vi "RTK-Make Child.vi"(1 "error in (no error)":errorcluster, 2 "Window Number":i32, 3 "Name of Parent Panel":string) -> (0 "error out":errorcluster)   [LabVIEW 2021]
doc: "Developer: Wayne Lootsma\nDate: 01/08/2003\nDescription:\nVi from NIs website for making an IMAQ window a child window, works only on Windows systems. Here is the original text:\nIMAQ MakeChild will allow you to embed your IMAQ Vision display into any vi's Front Panel.\n\nIt is okay to use IMAQ WindMove, IMAQ WindSize, IMAQ WindSetup, etc to define properties of the child window before calling this function. Doing so will allow you to customize the look and feel of your user interface.\n\nParent Panel Name is the name of the vi into which the IMAQ Vision window is to be embedded. This vi must be loaded into memory. \n\nWindow Number is the IMAQ Vision window number of the window which is to be made a child. This number is specified in IMAQ Create. \n\n\nDialog Panel: False\nGUI Panel: False\n\nDLL Description:\nInterface with a window for an IMAQ window.\n\nParty's Responsible: Microsoft Corp.\nDLL Filename: User32.dll\nDLL Location: C:\\Windows\\System\nProduct Name, Compiler and Version Number: Microsoft Visual C++, C Compiler V 2.0\nOperating System: Windows NT, 2000.\nLast Date Modified: 03/26/2003"
uses:
  User32.dll
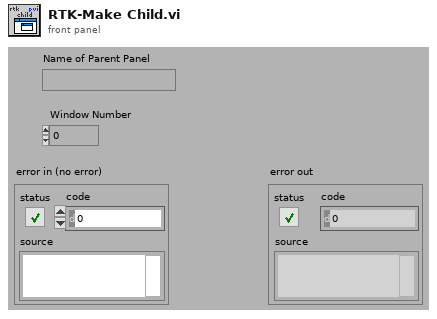
[diagram p1: front panel]
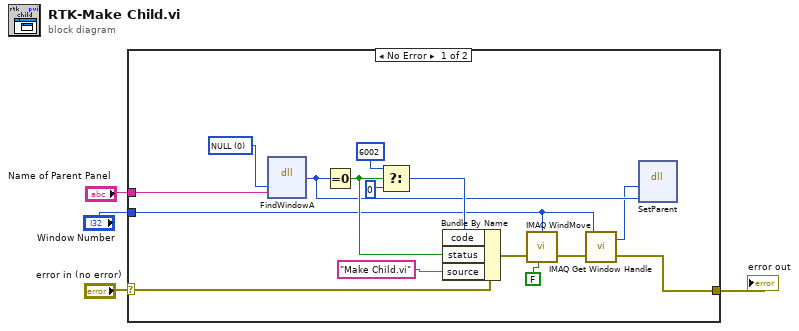
[diagram p0: block diagram]
diagram:
  n1 = case shown="No Error" "error in (no error)" {
    selector: "error in (no error)" -> [w7 w20]
    tunnel: [w8 w20] -> w4
    tunnel: "Name of Parent Panel" -> [w6 _]
    tunnel: "Window Number" -> [w5 _]
    frame No Error {
      w14 = 0 items=["NULL"]
      n2 = dll-call lib="user32.dll" fn="FindWindowA" label="FindWindow"("lpszClassName"=w14, "lpszWindowName"=w6) -> ("hWnd"=w13:u32)  [unwired: 5 in, 2 out]
      n3 = Equal To 0?(x=w13) -> (x = 0?=w18:bool)
      n4 = Select(t=6002, s=w18, f=0) -> (s? t:f=w19:i32)
      n5 = Bundle By Name(cluster=w7, "code"=w19, "status"=w18, "source"="Make Child.vi") -> (w11:errorcluster)
      n6 = call "IMAQ WindMove"("Window Number (0...15)"=w5, "Get/Set Status? (Set)"=FALSE, "error in (no error)"=w11) -> ("error out"=w10:errorcluster)  [unwired: 2 in, 1 out]
      n7 = call "IMAQ Get Window Handle"("error in (no error)"=w10, "Window Number"=w5) -> ("error out"=w8:errorcluster, "Handle"=w12:u64)
      n8 = dll-call lib="user32.dll" fn="SetParent"("Child"=w12, "NewParent"=w13) -> ()  [unwired: 6 in, 2 out]
    }
    frame Error {
    }
  }
  "error out" <- w4
